vi "Scan engine status.vi"(0 "XY Graph in":cluster{"X":dbl, "Y":dbl}[](graph), 1 "Actions":T2=enum."Clear", 5 "Current Position in":cluster{"X":dbl, "Y":dbl}, 9 "Current state in":T1=enum."Init(GPU FFT)", 11 "Error In":errorcluster, 12 "image plane":dbl format="%#_13g", 13 "slice plane":dbl format="%#_13g") -> (2 "slice plane out":dbl, 3 "image plane out":dbl, 4 "XY Graph out":cluster{"X":dbl, "Y":dbl}[](graph), 6 "Current Position out":cluster{"X":dbl, "Y":dbl}, 10 "Current state out":T1=enum."Init(GPU FFT)", 15 "Error Out":errorcluster)   [LabVIEW 2018]
uses:
  Controls/Go Scan Actions.ctl
  Controls/FGV Actions.ctl
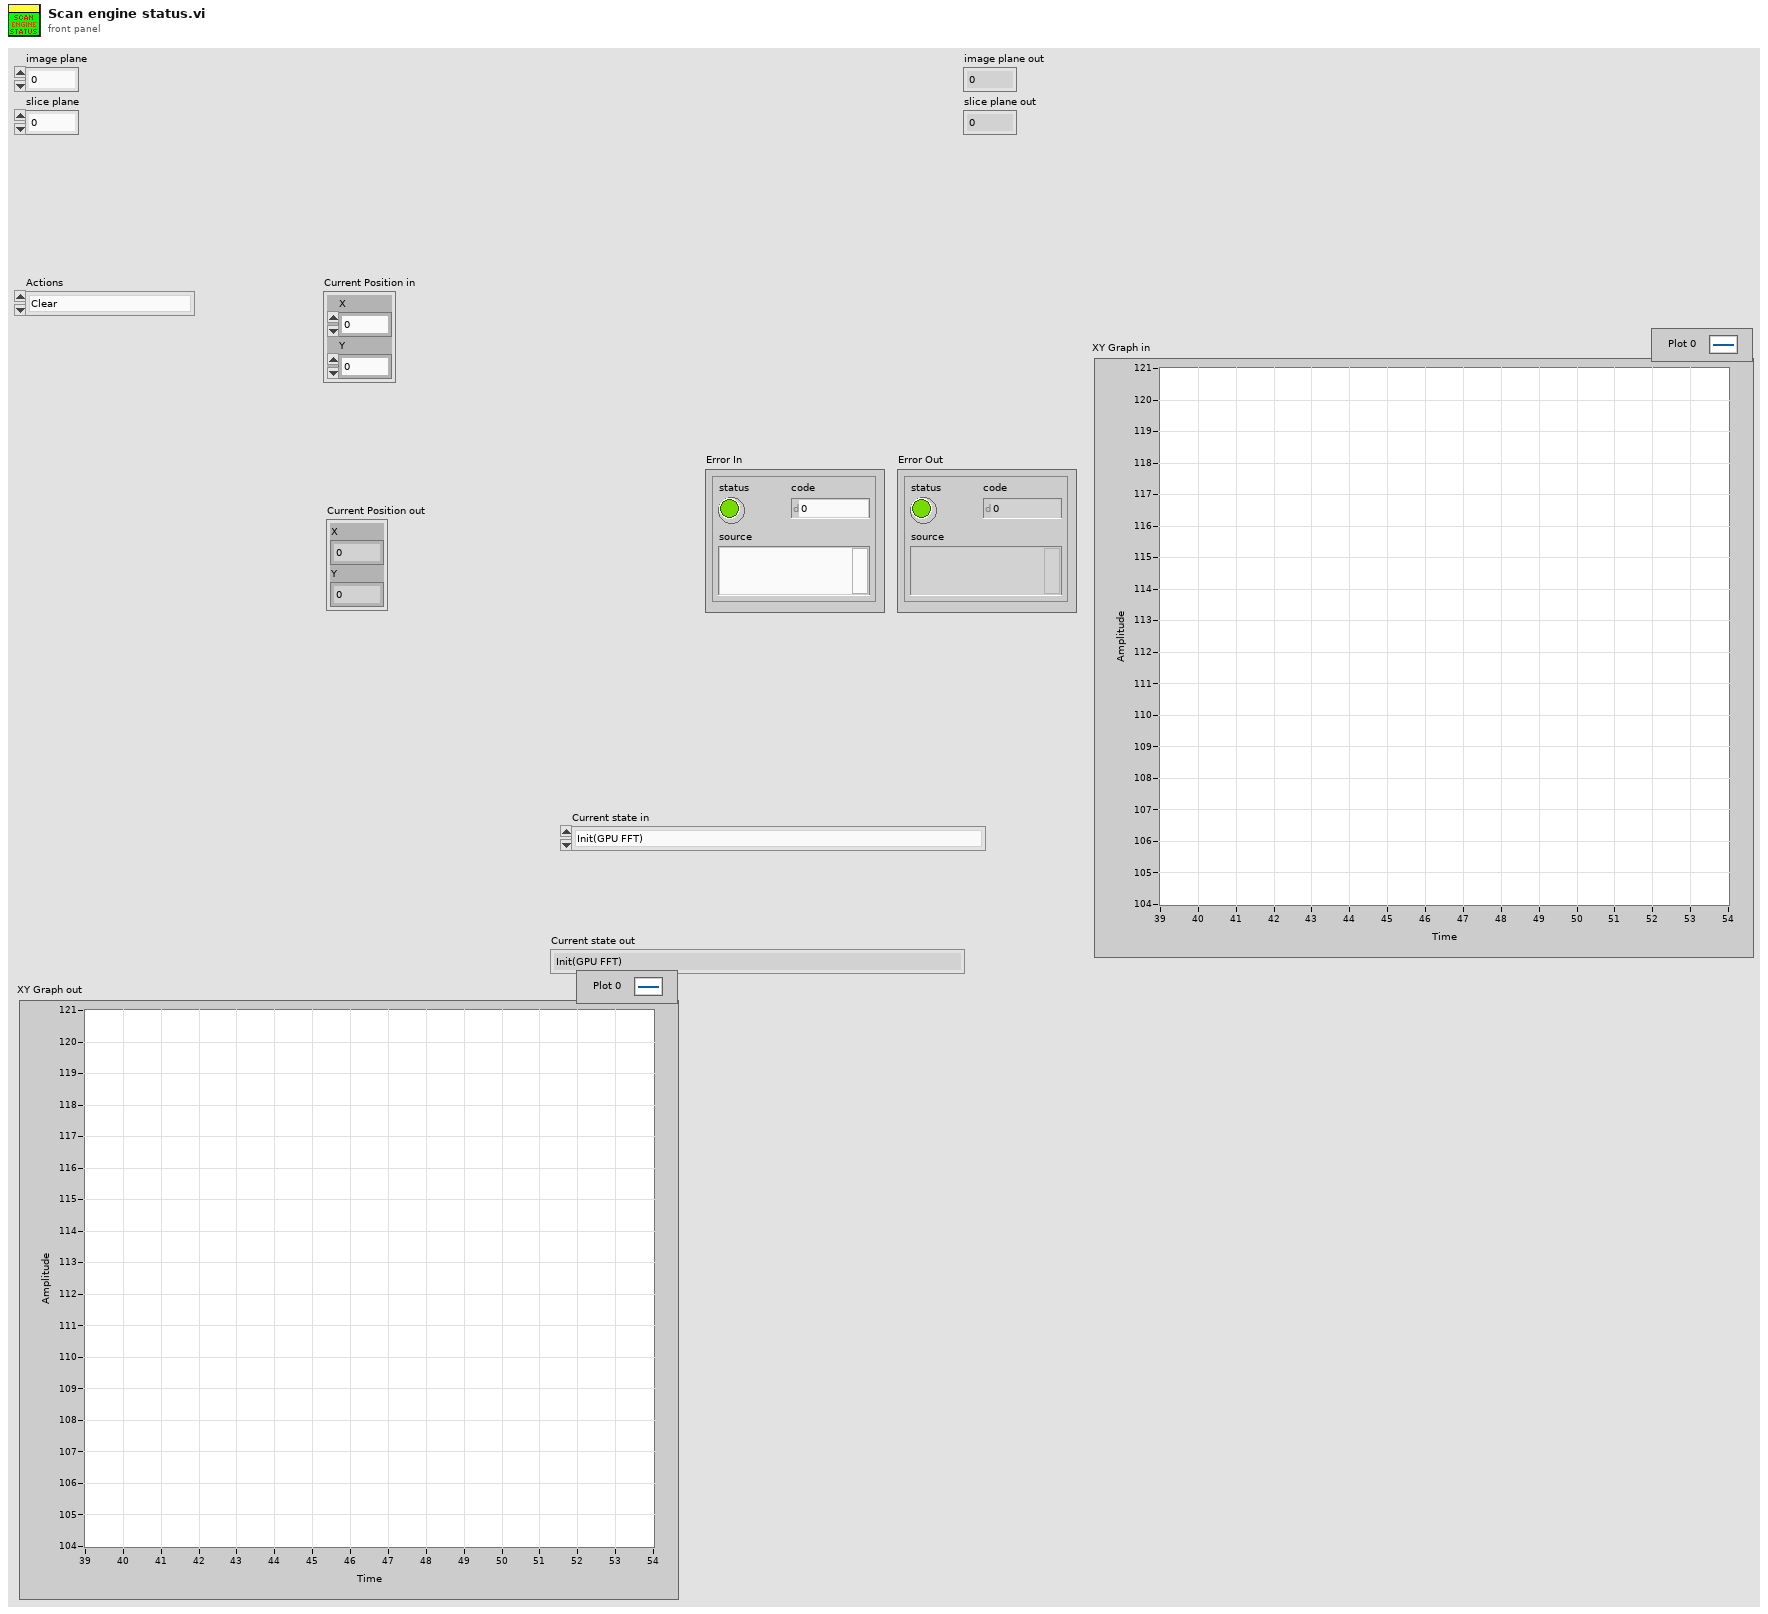
[diagram p1: front panel]
types:
  T1 = typedef "Go Scan Actions.ctl" = enum16{"Init(ThorOCT Spatial)", "Init(ThorOCT Spectral)", "Init(GPU FFT)", "Init(Alazar FFT)", "Init Scan Head(ThorOCT Spectral)", "Init Scan Head(ThorOCT Spatial)", "Init Scan Head", "Init Table Stage", "Init Vibratome", "Generate Mosaic", "Generate Z Position", "Go to Image Z", "Go Image Home", "Go Mosaic", "Acquire Image(ThorOCT Spatial)", "Acquire Image(ThorOCT Spectral)", "Acquire Image(GPU FFT)", "Acquire Image(Alazar FFT)", "Go Vibratome", "Slice", "Finished(ThorOCT)", "Finished", "Init(Alazar Spectral)", "Go Vibratome3"}
  T2 = typedef "FGV Actions.ctl" = enum16{"Init", "Set", "Get", "Clear"}
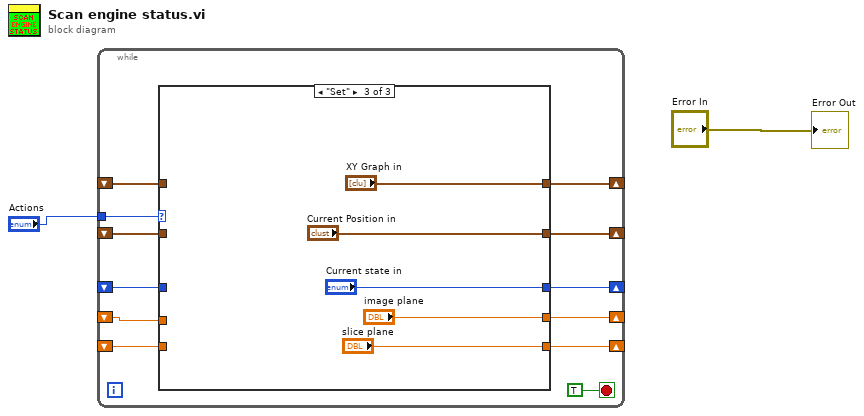
[diagram p0: block diagram]
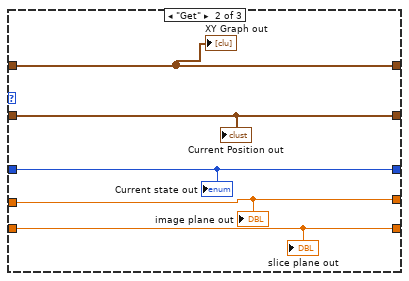
[diagram p3: hidden frame]
diagram:
  n1 = while {
    shift-right: [w14] -> _
    shift-left: _ -> [w10]
    shift-right: [w13] -> _
    shift-left: _ -> [w9]
    shift-right: [w12] -> _
    shift-left: _ -> [w8]
    tunnel: "Actions" -> [w11]
    shift-right: [w6] -> _
    shift-left: _ -> [w4]
    shift-right: [w5] -> _
    shift-left: _ -> [w3]
    stop <- TRUE stop-if-true
    n2 = case shown="\"Set\"" w11 {
      tunnel: [_ w17 "XY Graph in"] -> w14
      tunnel: [_ w19 "Current Position in"] -> w13
      tunnel: [_ w18 "Current state in"] -> w12
      tunnel: w10 -> [_ w17 _]
      tunnel: w9 -> [_ w19 _]
      tunnel: w8 -> [_ w18 _]
      tunnel: [_ w16 "image plane"] -> w6
      tunnel: [_ w15 "slice plane"] -> w5
      tunnel: w4 -> [_ w16 _]
      tunnel: w3 -> [_ w15 _]
      frame "Init", Default {
      }
      frame "Get" {
        "Current Position out" <- w19
        "Current state out" <- w18
        "XY Graph out" <- w17
        "image plane out" <- w16
        "slice plane out" <- w15
      }
      frame "Set" {
      }
    }
  }
  "Error Out" <- "Error In"
